vi "Reaction_space.vi"(9 "Relative velocity m/s":dbl, 10 "Obstacle Y":dbl, 11 "Obstacle X":dbl) -> ()   [LabVIEW 2020]
panel:
  out "Time to react":string
  out "Speed":dbl format="%#_6p km/h"
  out "Reaction space":cluster{dbl[], dbl[]}[](graph)
  out "clothoid end angle":dbl
  out "clothoid end distance":dbl
  in  "ds":dbl
  out "Clothoid parameter":dbl
  out "Clothoid length":dbl
  out "Max curve radius":dbl
  out "Braking distance":dbl
  in  "Friction coefficient":dbl
  out "Car speed m/s":dbl
  in  "Car speed km/h":dbl
  in  "Y limit":dbl
  in  "Car response time":dbl
  in  "Reaction time":dbl
  in  "Car width":dbl
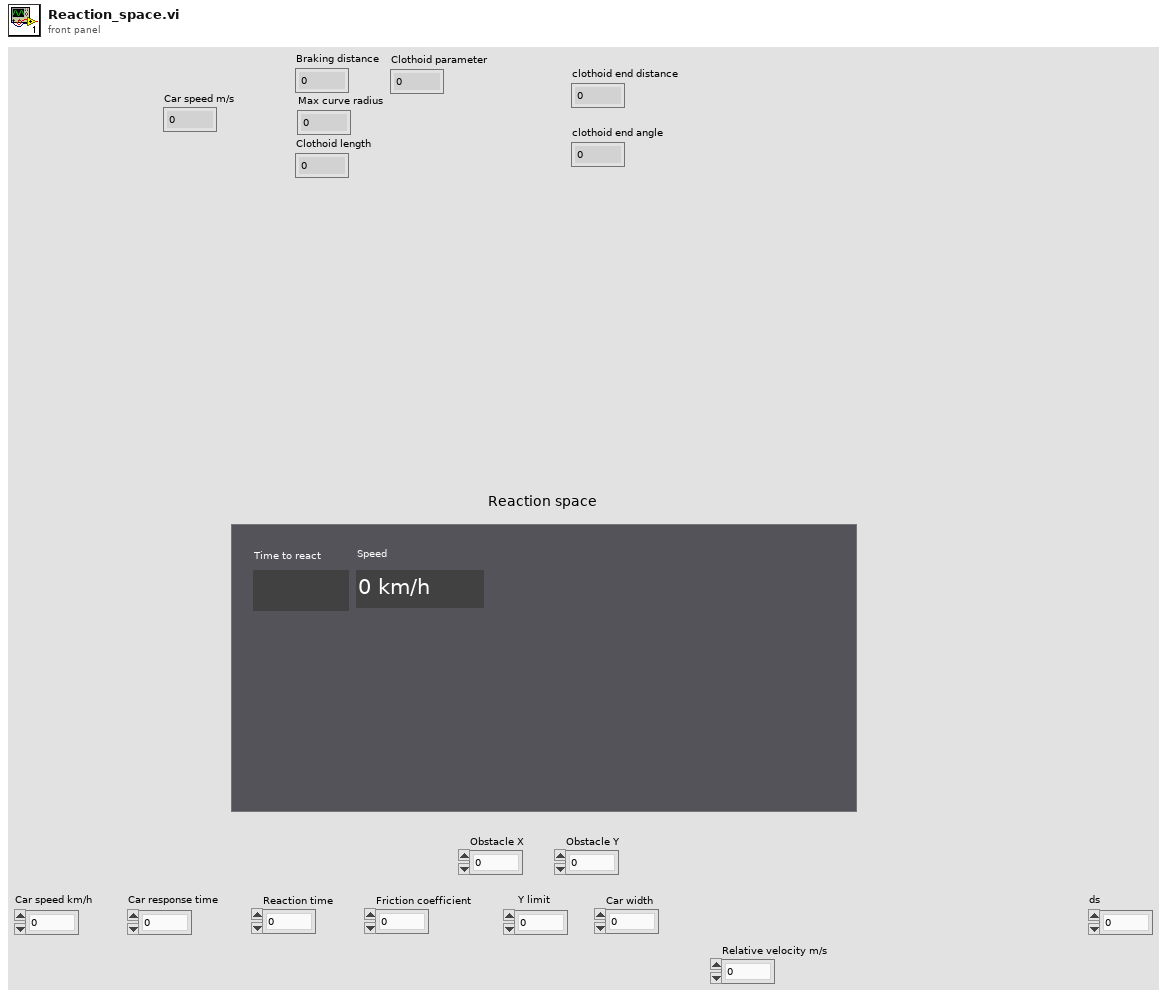
[diagram p1: front panel]
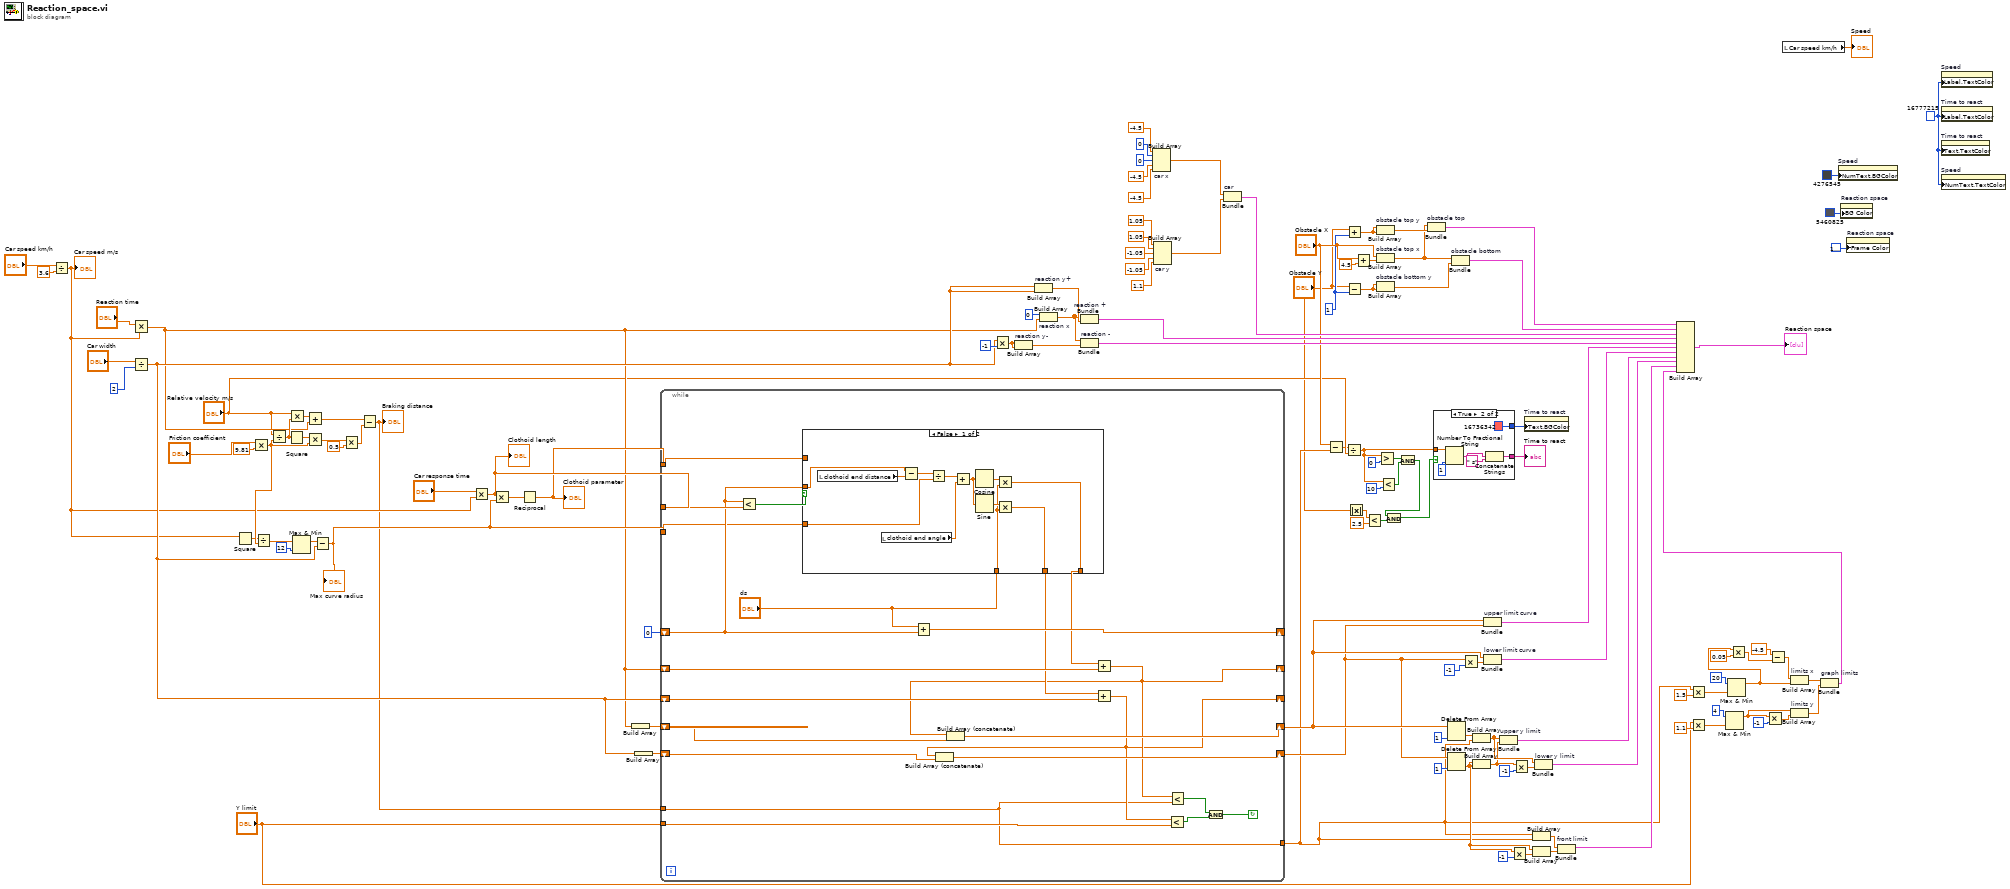
[diagram p0: block diagram]
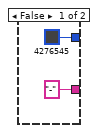
[diagram p2: hidden frame]
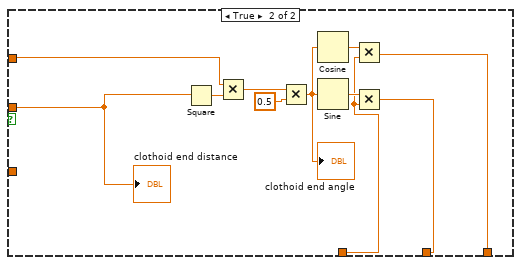
[diagram p3: hidden frame]
diagram:
  w12 = u32 16777215
  w46 = 1
  n1 = Divide(x="Car speed km/h", y=3.6) -> (x/y=w36:dbl)
  "Car speed m/s" <- w36
  n2 = Multiply(x="Reaction time", y=w36) -> (x*y=w33:dbl)
  n3 = Divide(x="Car width", y=2) -> (x/y=w88:dbl)
  n4 = Square(x=w36) -> (x^2=w101:dbl)
  n5 = Multiply(x="Friction coefficient", y=9.81) -> (x*y=w102:dbl)
  n6 = Divide(x=w101, y=w102) -> (x/y=w99:dbl)
  n7 = Divide(x="Relative velocity m/s", y=w102) -> (x/y=w107:dbl)
  n8 = Square(x=w107) -> (x^2=w106:dbl)
  n9 = Multiply(x="Relative velocity m/s", y=w107) -> (x*y=w109:dbl)
  n10 = Max & Min(x=w99, y=12) -> (max(x,y)=w100:dbl)  [unwired: 1 out]
  n11 = Add(x=w109, y=w33) -> (x+y=w108:dbl)
  n12 = Multiply(x=w106, y=w102) -> (x*y=w105:dbl)
  n13 = Subtract(x=w100, y=w88) -> (x-y=w35:dbl)
  "Max curve radius" <- w35
  n14 = Multiply(x=w105, y=0.5) -> (x*y=w103:dbl)
  n15 = Subtract(x=w108, y=w103) -> (x-y=w34:dbl)
  "Braking distance" <- w34
  n16 = Multiply(x="Car response time", y=w36) -> (x*y=w93:dbl)
  "Clothoid length" <- w93
  n17 = Multiply(x=w93, y=w35) -> (x*y=w96:dbl)
  n18 = Reciprocal(x=w96) -> (1/x=w37:dbl)
  "Clothoid parameter" <- w37
  n19 = Build Array(w33) -> (w90:dbl[])
  n20 = Build Array(w88) -> (w89:dbl[])
  n21 = while "s" {
    shift-right: [w129] -> _
    shift-left: w33 -> [w142]
    shift-right: [w128] -> _
    shift-left: w88 -> [w143]
    shift-right: [w141] -> _
    shift-left: 0 -> [w135]
    tunnel: w93 -> [w140]
    tunnel: w35 -> [w134]
    shift-right: [w130] -> w84
    shift-left: w89 -> [w131]
    shift-right: [w132] -> w87
    shift-left: w90 -> [w133]
    tunnel: w37 -> [w127]
    tunnel: "Y limit" -> [w126]
    tunnel: [w125] -> w8
    tunnel: w34 -> [w125]
    stop <- w144 continue-if-true
    n22 = Less?(x=w135, y=w140) -> (x < y?=w139:bool)
    n23 = case shown="False" w139 {
      tunnel: w135 -> [w158 w160]
      tunnel: "ds" -> [w149 w164]
      tunnel: [w148 w163] -> w137
      tunnel: [w147 w162] -> w136
      tunnel: w134 -> [w155 _]
      tunnel: w127 -> [_ w159]
      frame False {
        n24 = local read "clothoid end distance"() -> (w157:dbl)
        n25 = local read "clothoid end angle"() -> (w154:dbl)
        n26 = Subtract(x=w158, y=w157) -> (x-y=w156:dbl)
        n27 = Divide(x=w156, y=w155) -> (x/y=w153:dbl)
        n28 = Add(x=w153, y=w154) -> (x+y=w152:dbl)
        n29 = Cosine(x=w152) -> (cos(x)=w151:dbl)
        n30 = Sine(x=w152) -> (sin(x)=w150:dbl)
        n31 = Multiply(x=w151, y=w149) -> (x*y=w148:dbl)
        n32 = Multiply(x=w150, y=w149) -> (x*y=w147:dbl)
      }
      frame True {
        n33 = Square(x=w160) -> (x^2=w169:dbl)
        n34 = Multiply(x=w159, y=w169) -> (x*y=w168:dbl)
        n35 = Multiply(x=w168, y=0.5) -> (x*y=w161:dbl)
        "clothoid end angle" <- w161
        n36 = Cosine(x=w161) -> (cos(x)=w166:dbl)
        n37 = Sine(x=w161) -> (sin(x)=w165:dbl)
        n38 = Multiply(x=w166, y=w164) -> (x*y=w163:dbl)
        n39 = Multiply(x=w165, y=w164) -> (x*y=w162:dbl)
        "clothoid end distance" <- w160
      }
    }
    n40 = Add(x="ds", y=w135) -> (x+y=w141:dbl)
    n41 = Add(x=w137, y=w142) -> (x+y=w129:dbl)
    n42 = Build Array (concatenate)(w129, w133) -> (w132:dbl[])
    n43 = Add(x=w136, y=w143) -> (x+y=w128:dbl)
    n44 = Build Array (concatenate)(w128, w131) -> (w130:dbl[])
    n45 = Less?(x=w128, y=w126) -> (x < y?=w146:bool)
    n46 = Less?(x=w129, y=w125) -> (x < y?=w145:bool)
    n47 = And(x=w145, y=w146) -> (x .and. y?=w144:bool)
  }
  n48 = Multiply(x=w88, y=-1) -> (x*y=w120:dbl)
  n49 = Build Array "reaction y-"(w120, w120) -> (w118:dbl[])
  n50 = Build Array "reaction y+"(w88, w88) -> (w119:dbl[])
  n51 = Build Array "reaction x"(0, w33) -> (w117:dbl[])
  n52 = Bundle "reaction +"(w117, w119) -> (w116:cluster{dbl[], dbl[]})  [unwired: 1 in]
  n53 = Bundle "reaction -"(w117, w118) -> (w115:cluster{dbl[], dbl[]})  [unwired: 1 in]
  n54 = Build Array "car x"(-4.5, 0, 0, -4.5, -4.5) -> (w62:dbl[])
  n55 = Build Array "car y"(1.05, 1.05, -1.05, -1.05, 1.1) -> (w61:dbl[])
  n56 = Bundle "car"(w62, w61) -> (w60:cluster{dbl[], dbl[]})  [unwired: 1 in]
  n57 = Subtract(x="Obstacle X", y=w8) -> (x-y=w18:dbl)
  n58 = Divide(x=w18, y="Relative velocity m/s") -> (x/y=w13:dbl)
  n59 = Add(x="Obstacle Y", y=w46) -> (x+y=w54:dbl)
  n60 = Subtract(x="Obstacle Y", y=w46) -> (x-y=w50:dbl)
  n61 = Absolute Value(x="Obstacle Y") -> (abs(x)=w6:dbl)
  n62 = Add(x="Obstacle X", y=4.5) -> (x+y=w56:dbl)
  n63 = Less?(x=w6, y=2.5) -> (x < y?=w2:bool)
  n64 = Build Array "obstacle top y"(w54, w54) -> (w55:dbl[])
  n65 = Build Array "obstacle top x"("Obstacle X", w56) -> (w51:dbl[])
  n66 = Build Array "obstacle bottom y"(w50, w50) -> (w53:dbl[])
  n67 = Greater?(x=w13, y=0) -> (0:w14:bool)
  n68 = Less?(x=w13, y=10) -> (x < y?=w15:bool)
  n69 = And(x=w14, y=w15) -> (x .and. y?=w3:bool)
  n70 = And(x=w3, y=w2) -> (x .and. y?=w4:bool)
  n71 = Bundle "obstacle top"(w51, w55) -> (w52:cluster{dbl[], dbl[]})  [unwired: 1 in]
  n72 = case shown="True" w4 {
    tunnel: ["-" w177] -> w11
    tunnel: w13 -> [_ w174]
    tunnel: [u32 4276545 u32 16736342] -> w10
    frame False {
    }
    frame True {
      n73 = Number To Fractional String(number=w174, precision (6)=1) -> (F-format string=w173:string)  [unwired: 2 in]
      n74 = Concatenate Strings(w173, " s") -> (w177:string)
    }
  }
  "Time to react" <- w11
  n75 = Delete From Array(array=w87, index=1) -> (deleted portion=w9:dbl)  [unwired: 1 in, 1 out]
  n76 = Delete From Array(array=w84, index=1) -> (deleted portion=w74:dbl)  [unwired: 1 in, 1 out]
  n77 = Bundle "obstacle bottom"(w51, w53) -> (w49:cluster{dbl[], dbl[]})  [unwired: 1 in]
  n78 = Multiply(x=w84, y=-1) -> (x*y=w92:dbl[])
  n79 = Build Array(w9, w8) -> (w82:dbl[])
  n80 = Build Array(w74, w74) -> (w79:dbl[])
  n81 = Bundle "upper limit curve"(w87, w84) -> (w95:cluster{dbl[], dbl[]})  [unwired: 1 in]
  n82 = Bundle "lower limit curve"(w87, w92) -> (w91:cluster{dbl[], dbl[]})  [unwired: 1 in]
  n83 = Bundle "upper y limit"(w82, w79) -> (w78:cluster{dbl[], dbl[]})  [unwired: 1 in]
  n84 = Multiply(x=w74, y=-1) -> (x*y=w76:dbl)
  n85 = Multiply(x=w79, y=-1) -> (x*y=w80:dbl[])
  n86 = property on="Time to react" class="Str"("Text.BGColor"=w10) -> ()  [unwired: 2 in, 2 out]
  n87 = Build Array(w8, w8) -> (w73:dbl[])
  n88 = Build Array(w74, w76) -> (w72:dbl[])
  n89 = Bundle "lower y limit"(w82, w80) -> (w77:cluster{dbl[], dbl[]})  [unwired: 1 in]
  n90 = Bundle "front limit"(w73, w72) -> (w71:cluster{dbl[], dbl[]})  [unwired: 1 in]
  n91 = Multiply(x=w8, y=1.5) -> (x*y=w38:dbl)
  n92 = Multiply(x="Y limit", y=1.1) -> (x*y=w28:dbl)
  n93 = Max & Min(x=4, y=w28) -> (max(x,y)=w25:dbl)  [unwired: 1 out]
  n94 = Max & Min(x=20, y=w38) -> (max(x,y)=w7:dbl)  [unwired: 1 out]
  n95 = Multiply(x=w7, y=0.05) -> (x*y=w41:dbl)
  n96 = Multiply(x=w25, y=-1) -> (x*y=w24:dbl)
  n97 = Subtract(x=-4.5, y=w41) -> (x-y=w31:dbl)
  n98 = local read "Car speed km/h"() -> (→"Speed":dbl)
  n99 = Build Array "limits x"(w31, w7) -> (w22:dbl[])
  n100 = Build Array "limits y"(w25, w24) -> (w23:dbl[])
  n101 = Bundle "graph limits"(w22, w23) -> (w21:cluster{dbl[], dbl[]})  [unwired: 1 in]
  n102 = Build Array(w52, w49, w60, w116, w115, w95, w91, w78, w77, w71, w21) -> (→"Reaction space":cluster{dbl[], dbl[]}[])
  n103 = property on="Speed" class="DigNum (strict)"("NumText.BGColor"=u32 4276545) -> ()  [unwired: 2 in, 2 out]
  n104 = property on="Reaction space" class="XYGraph (strict)"("BG Color"=u32 5460825) -> ()  [unwired: 2 in, 2 out]
  n105 = property on="Reaction space" class="XYGraph (strict)"("Frame Color"=u32 16777216) -> ()  [unwired: 2 in, 2 out]
  n106 = property on="Speed" class="DigNum (strict)"("Label.TextColor"=w12) -> ()  [unwired: 2 in, 2 out]
  n107 = property on="Time to react" class="Str"("Label.TextColor"=w12) -> ()  [unwired: 2 in, 2 out]
  n108 = property on="Time to react" class="Str"("Text.TextColor"=w12) -> ()  [unwired: 2 in, 2 out]
  n109 = property on="Speed" class="DigNum (strict)"("NumText.TextColor"=w12) -> ()  [unwired: 2 in, 2 out]
